vi "Read N Registers.vi"(8 "Error In":errorcluster, 10 "Addresses":u8[](array[numeric]), 11 "Adept Config":T1) -> (0 "Error Out":errorcluster, 2 "Data":u8[](array[numeric]), 3 "Adept Config":T1)   [LabVIEW 2011, in "LVH-Adept.lvlib"]
uses:
  Private/Type Defs/Device Config.ctl
  Private/Type Defs/Status.ctl
  LVH-Adept.lvlib
  Private/DEPP/DEPP.lvlib
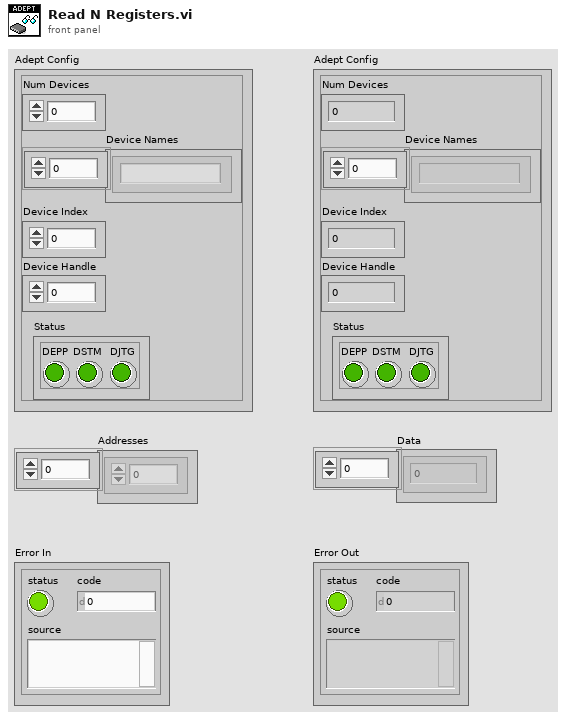
[diagram p1: front panel]
types:
  T1 = typedef "LVH-Adept.lvlib/Device Config.ctl" = cluster{"Num Devices":i32, "Device Names":string[], "Device Index":u16, "Device Handle":u32, "Status":T2}
  T2 = typedef "LVH-Adept.lvlib/Status.ctl" = cluster{"DEPP":bool, "DSTM":bool, "DJTG":bool}
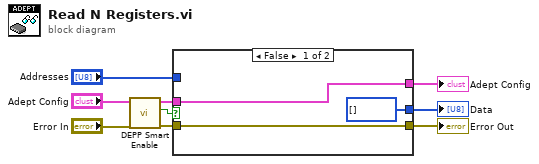
[diagram p0: block diagram]
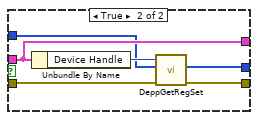
[diagram p2: hidden frame]
diagram:
  n1 = call "DEPP Smart Enable.vi"("Error In"="Error In", "Adept Config"="Adept Config") -> ("Error Out"=w7:errorcluster, "Success?"=w6:bool, "Adept Config"=w4:T1)  [unwired: 7 in]
  n2 = case shown="False" w6 {
    tunnel: w7 -> [w12 w15]
    tunnel: w4 -> [w11 w18]
    tunnel: [w12 w16] -> w5
    tunnel: [u8[] [] ("Data") w14] -> w2
    tunnel: [w11 w18] -> w3
    tunnel: "Addresses" -> [_ w13]
    frame False {
    }
    frame True {
      n3 = Unbundle By Name(w18) -> ("Device Handle"=w17:u32)
      n4 = call "DeppGetRegSet.vi"("Error In"=w15, "Addresses"=w13, "Device Handle"=w17) -> ("Error Out"=w16:errorcluster, "Data"=w14:u8[])  [unwired: 6 in, 1 out]
    }
  }
  "Error Out" <- w5
  "Adept Config" <- w3
  "Data" <- w2
